vi "UnregisterForDiagPackets.vi"(0 "Event Metadata":T1, 3 "error in (no error)":errorcluster) -> (10 "error out":errorcluster)   [LabVIEW 2020, in "Aerotech.lvlib"]
uses:
  Aerotech.lvlib
  AxisDiagPacket.ctl
  ControllerDiagPacket.ctl
  C:/Users/HEP/Documents/GitHub/UCSB-Gantry-HEP/Drivers/Aerotech A3200/Bin/Aerotech.A3200.LabVIEW.dll
  UCSB-Gantry-HEP/Drivers/Aerotech A3200/Bin/Aerotech.A3200.LabVIEW.dll
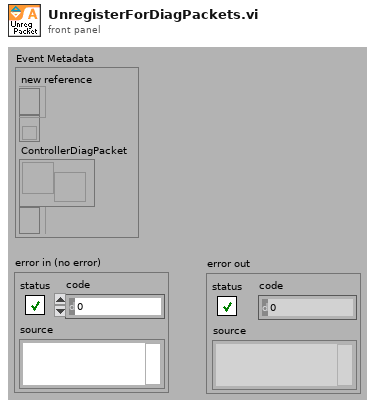
[diagram p1: front panel]
types:
  T1 = cluster{"new reference":refnum<k24>, "Event Callback":refnum<k27>, "ControllerDiagPacket":refnum<user-event>, "Event Registration Refnum":refnum<event-registration>}
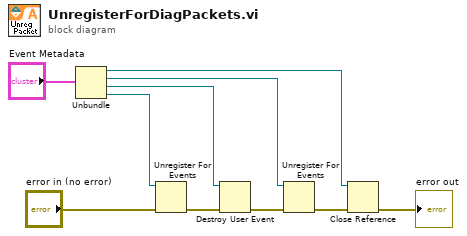
[diagram p0: block diagram]
diagram:
  n1 = Unbundle("Event Metadata") -> ("new reference"=w5:refnum<k24>, "Event Callback"=w4:refnum<k27>, "ControllerDiagPacket"=w3:refnum<user-event>, "Event Registration Refnum"=w2:refnum<event-registration>)
  n2 = Unregister For Events(event registration refnum=w2, error in="error in (no error)") -> (error out=w9:errorcluster)
  n3 = Destroy User Event(user event=w3, error in=w9) -> (error out=w8:errorcluster)
  n4 = Unregister For Events(event registration refnum=w4, error in=w8) -> (error out=w7:errorcluster)
  n5 = Close Reference(reference=w5, error in (no error)=w7) -> (error out=→"error out":errorcluster)
